vi "2086发送.vi"() -> ()   [LabVIEW 2016, in "数据传输系统-03.lvlib"]
uses:
  <vilib>/Utility/config.llb/Write Key (String).vi
  <vilib>/Utility/config.llb/Read Key (String).vi
  <vilib>/Utility/config.llb/NI_LVConfig.lvlib
panel:
  out "数据发送起始时间":timestamp format="%<%.3X\n%Y/%m/%d>T"
  out "数据拆分":bool
  in  "设备类型":string(combo)="010200"
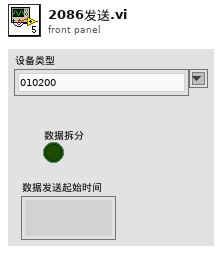
[diagram p1: front panel]
types:
  T1 = cluster{"CODMn":string, "CODCr":string, "DO":string, "铜":string, "PH":string, "氨氮":string, "比电导率":string, "水温":string, "COD":string, "浊度":string, "总氮":string, "总磷":string, "叶绿素a":string, "藻密度":string, "水位":string, "流速":string, "方向":string, "瞬时流量":string, "累积流量":string, "正累积流量":string, "负累积流量":string, "亚硝酸盐":string, "硫化物":string, "ORP":string, "铅":string, "镉":string, "锌":string, "镍":string, "锰":string, "汞":string, "气温":string, "气压":string, "风速":string, "风向":string, "空气温度":string, "相对湿度":string, "分钟雨量":string, "小时雨量":string, "日雨量":string, "累积雨量":string, "盐度":string, "磷酸盐":string, "硝氮":string, "氟化物":string, "挥发酚":string, "氯化物":string, "蓝绿藻":string, "余氯":string, "综合生物毒性":string, "艏向":string, "横摇":string, "纵摇":string, "分层标志":string, "层状态1":string, "层状态2":string, "水平平均流速":string, "流向":string, "北向流速分量":string, "东向流速分量":string, "垂直流速分量":string, "最大波高":string, "最大波周期":string, "1/10波高":string, "1/10波周期":string, "有效波高":string, "有效波周期":string, "平均波高":string, "平均波周期":string, "波向":string, "波个数":string, "水深":string, "X轴流速":string, "Y轴流速":string, "信号强度":string, "电压":string, "悬浮物":string}
  T2 = cluster{"QN":string, "ST":string, "CN":string, "PW":string, "MN":string, "FLAG":string, "PNUM":string, "PNO":string, "CP":string}
  T3 = typedef "LVComboBoxStrsAndValuesArrayTypeDef.ctl" = cluster{"String":string, "Value":string}[]
  T4 = typedef "数据传输系统-03.lvlib/应用环境.ctl" = enum16{"STD", "GB212", "婉仪平台"}
  T5 = cluster{"setini":string, "sysini":string, "hechaini":string, "actualwrite":string, "actualread":string, "datasent":string, "反控命令信息队列":string, "反控与仪器交互":string}
  T6 = cluster{"time1":string, "time2":string, "time3":string, "time4":string, "time5":string, "time6":string, "time7":string, "time8":string, "time9":string, "time10":string, "time11":string, "time12":string, "time13":string, "time14":string, "time15":string, "time16":string, "time17":string, "time18":string, "time19":string, "time20":string, "time21":string, "time22":string, "time23":string, "time24":string, "time25":string, "time26":string, "time27":string, "time28":string, "time29":string, "time30":string, "time31":string, "time32":string, "time33":string, "time34":string, "time35":string, "time36":string, "time37":string, "time38":string, "time39":string, "time40":string, "time41":string, "time42":string, "time43":string, "time44":string, "time45":string, "time46":string, "time47":string, "time48":string, "time49":string, "time50":string, "time51":string, "time52":string, "time53":string, "time54":string, "time55":string, "time56":string, "time57":string, "time58":string, "time59":string, "time60":string, "time61":string, "time62":string, "time63":string, "time64":string, "time65":string, "time66":string, "time67":string, "time68":string, "time69":string, "time70":string, "time71":string, "time72":string, "time73":string, "time74":string, "time75":string, "time76":string}
  T7 = cluster{"水样数据索引[0]":string, "水样数据索引[1]":string, "水样数据索引[2]":string, "水样数据索引[3]":string, "水样数据索引[4]":string, "水样数据索引[5]":string, "水样数据索引[6]":string, "水样数据索引[7]":string, "水样数据索引[8]":string, "水样数据索引[9]":string, "水样数据索引[10]":string, "水样数据索引[11]":string, "水样数据索引[12]":string, "水样数据索引[13]":string, "水样数据索引[14]":string, "水样数据索引[15]":string, "水样数据索引[16]":string, "水样数据索引[17]":string, "水样数据索引[18]":string, "水样数据索引[19]":string, "水样数据索引[20]":string, "水样数据索引[21]":string, "水样数据索引[22]":string, "水样数据索引[23]":string, "水样数据索引[24]":string, "水样数据索引[25]":string, "水样数据索引[26]":string, "水样数据索引[27]":string, "水样数据索引[28]":string, "水样数据索引[29]":string, "水样数据索引[30]":string, "水样数据索引[31]":string, "水样数据索引[32]":string, "水样数据索引[33]":string, "水样数据索引[34]":string, "水样数据索引[35]":string, "水样数据索引[36]":string, "水样数据索引[37]":string, "水样数据索引[38]":string, "水样数据索引[39]":string, "水样数据索引[40]":string, "水样数据索引[41]":string, "水样数据索引[42]":string, "水样数据索引[43]":string, "水样数据索引[44]":string, "水样数据索引[45]":string, "水样数据索引[46]":string, "水样数据索引[47]":string, "水样数据索引[48]":string, "水样数据索引[49]":string, "水样数据索引[50]":string, "水样数据索引[51]":string, "水样数据索引[52]":string, "水样数据索引[53]":string, "水样数据索引[54]":string, "水样数据索引[55]":string, "水样数据索引[56]":string, "水样数据索引[57]":string, "水样数据索引[58]":string, "水样数据索引[59]":string, "水样数据索引[60]":string, "水样数据索引[61]":string, "水样数据索引[62]":string, "水样数据索引[63]":string, "水样数据索引[64]":string, "水样数据索引[65]":string, "水样数据索引[66]":string, "水样数据索引[67]":string, "水样数据索引[68]":string, "水样数据索引[69]":string, "水样数据索引[70]":string, "水样数据索引[71]":string, "水样数据索引[72]":string, "水样数据索引[73]":string, "水样数据索引[74]":string, "水样数据索引[75]":string}
  T8 = typedef "NI_LVConfig.lvlib/Config Data RefNum.ctl" = refnum<k1>
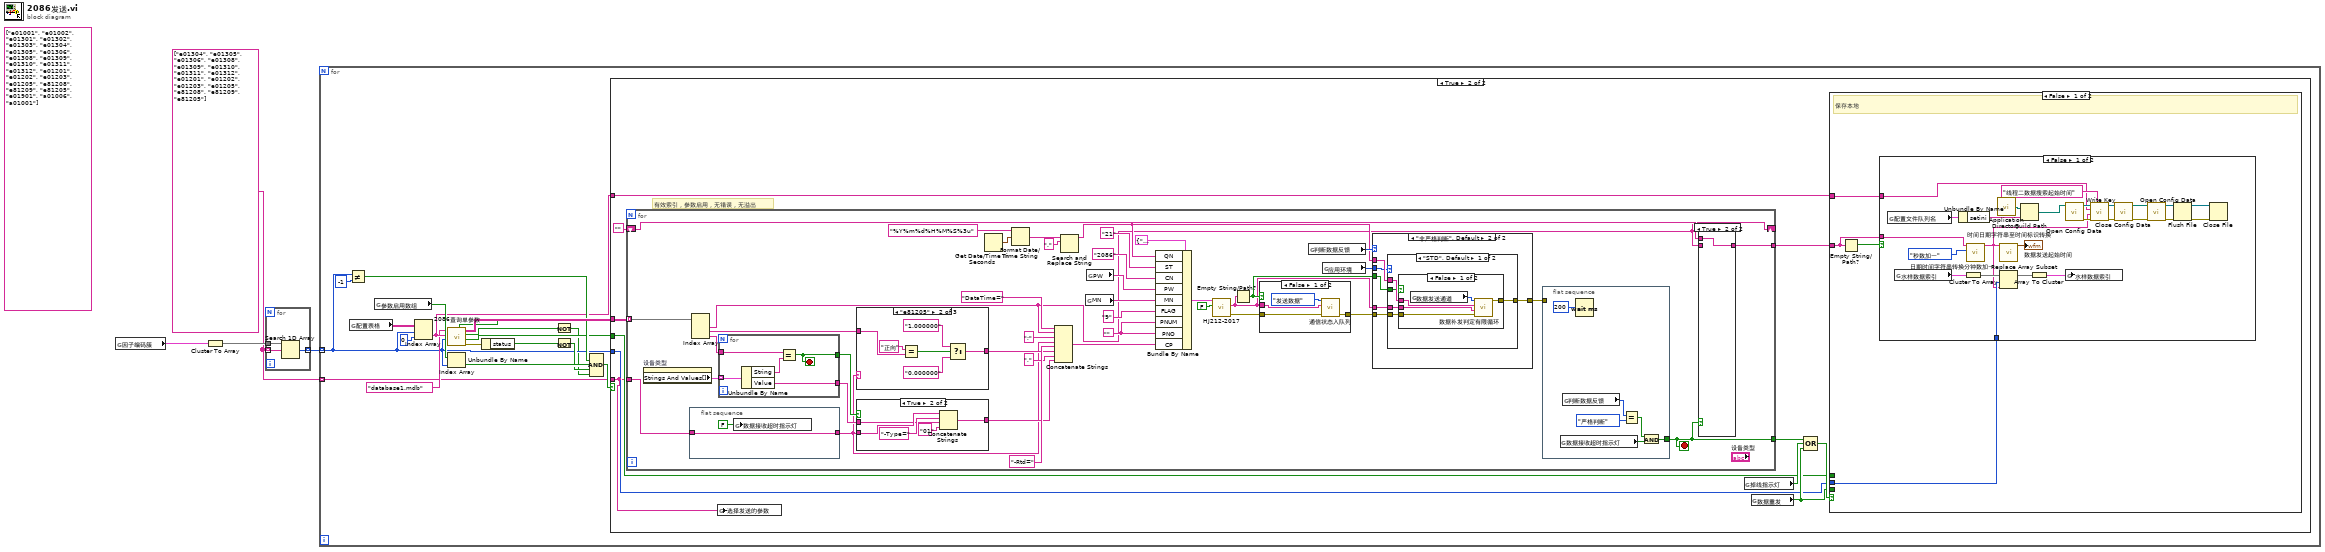
[diagram p0: block diagram]
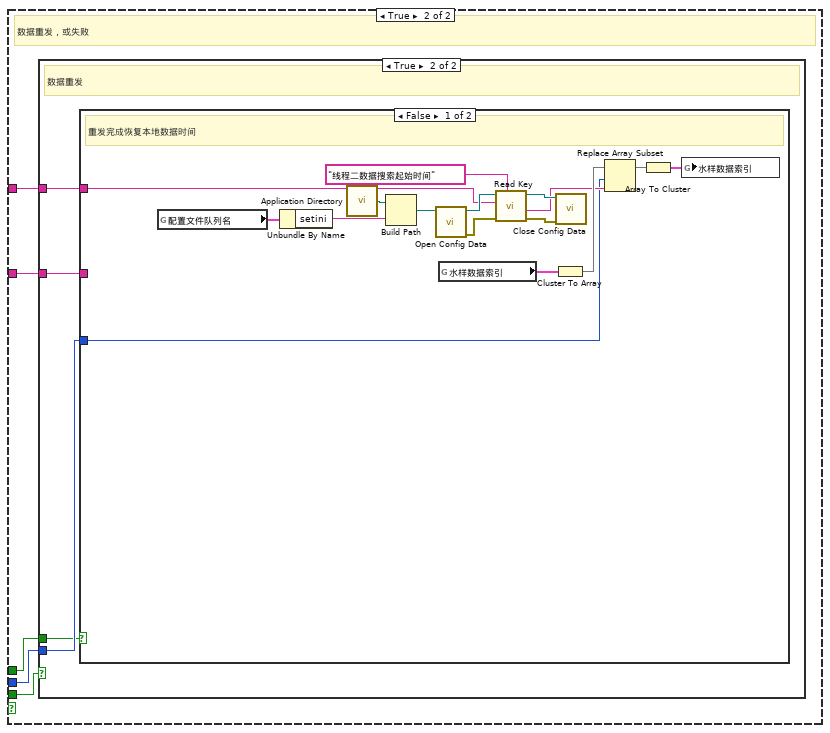
[diagram p4: hidden frame]
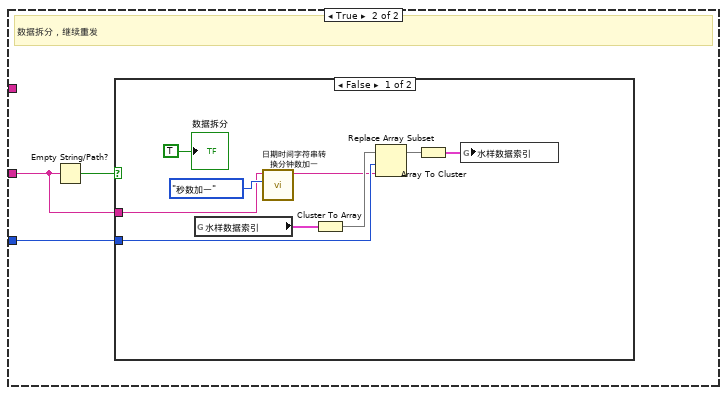
[diagram p6: hidden frame]
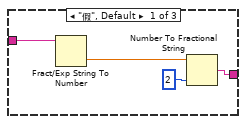
[diagram p9: hidden frame]
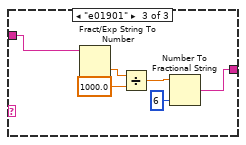
[diagram p10: hidden frame]
diagram:
  (unwired) string[] ["e01001", "e01002", "e01301", "e01302", "e01303", "e01304", "e01305", "e01306", "e01308", "e01309", "e01310", "e01311", "e01312", "e01201", "e01202", "e01203", "e01205", "e81208", "e81209", "e81205", "e01901", "a01006", "a01001"]
  w1 = string[] ["e01304", "e01305", "e01306", "e01308", "e01309", "e01310", "e01311", "e01312", "e01201", "e01202", "e01203", "e01205", "e81208", "e81209", "e81205"]
  n1 = global read "断电保存全局.vi" "因子编码簇"() -> (w4:T1)
  n2 = Cluster To Array(cluster=w4) -> (array=w3:string[])
  n3 = for {
    tunnel: w3 -> [w7]
    tunnel: w1 -> [w6] mode=indexing
    tunnel: [w5] -> w2 mode=indexing
    n4 = Search 1D Array(1D array=w7, element=w6) -> (index of element=w5:i32)  [unwired: 1 in]
  }
  n5 = for {
    tunnel: w2 -> [w11] mode=indexing
    tunnel: w1 -> [w10] mode=indexing
    n6 = Not Equal?(x=w11, y=-1) -> (x != y?=w21:bool)
    n7 = global read "断电保存全局.vi" "配置表格"() -> (w25:string[][])
    n8 = global read "断电保存全局.vi" "参数启用数组"() -> (w22:bool[])
    n9 = Index Array(array=w25, index (row)=w11, index (col)=0 ("y")) -> (element=w19:string)
    n10 = call "2086查询单参数.vi"("索引"=w11, "table"=w19, "database"="database1.mdb") -> ("error out"=w16:errorcluster, "拆分数据"=w17:bool, "database溢出"=w12:bool, "data"=w23:string[][], "有数据"=w8:bool)  [unwired: 4 in]
    n11 = Index Array(array=w22, index=w11) -> (element=w20:bool)
    n12 = Unbundle By Name(w16) -> ("status"=w15:bool)
    n13 = Not(x=w12) -> (.not. x?=w9:bool)
    n14 = Not(x=w15) -> (.not. x?=w14:bool)
    n15 = Compound Arithmetic op=AND ("复合运算")(w8, w21, w20, w14, w9) -> (w13:bool)
    n16 = case shown="True" w13 {
      tunnel: w23 -> [_ w37]
      tunnel: w10 -> [_ w27]
      tunnel: w19 -> [_ w32]
      tunnel: w11 -> [_ w31]
      tunnel: w17 -> [_ w30]
      frame False {
      }
      frame True {
        # "有效索引，参数启用，无错误，无溢出"
        n17 = for {
          tunnel: w37 -> [w104] mode=indexing
          tunnel: w27 -> [w106]
          tunnel: [w110] -> w36
          shift-right: [w105] -> _
          shift-left: "" -> [w109]
          tunnel: [w108] -> w29
          stop <- w110 stop-if-true
          w133 = ""
          n18 = property on="设备类型" class="CmbBox"() -> ("Strings And Values[]"=w126:T3)  [unwired: 2 in, 2 out]
          n19 = flat-sequence {
            tunnel: [w145] -> w107
            tunnel: w106 -> [w145]
            frame #0 {
              n20 = global write "全局 数据发送重叠.vi" "数据接收超时指示灯"(FALSE ("数据接收超时指示灯")) -> ()
            }
          }
          n21 = Index Array(array=w104) -> (element #1=w105:string, element #2=w112:string, element #3=w123:string)  [unwired: 3 in]
          n22 = for {
            tunnel: w126 -> [w200] mode=indexing
            tunnel: w123 -> [w198]
            tunnel: [w197] -> w124
            tunnel: [w196] -> w125
            stop <- w196 stop-if-true
            n23 = Unbundle By Name(w200) -> ("String"=w199:string, "Value"=w197:string)
            n24 = Equal?(x=w198, y=w199) -> (x = y?=w196:bool)
          }
          n25 = case shown="\"e81205\"" w107 {
            tunnel: w112 -> [w149 w157 w159]
            tunnel: [w148 w152 w158] -> w111
            frame "假", Default {
              n26 = Fract/Exp String To Number(string=w149) -> (number=w151:dbl)  [unwired: 3 in, 1 out]
              n27 = Number To Fractional String(number=w151, precision (6)=i16 2 ("精度(6)")) -> (F-format string=w148:string)  [unwired: 2 in]
            }
            frame "e81205" {
              n28 = Equal?(x="正向", y=w157) -> (x = y?=w155:bool)
              n29 = Select(t="1.000000" ("x"), s=w155, f="0.000000" ("x")) -> (s? t:f=w152:string)
            }
            frame "e01901" {
              n30 = Fract/Exp String To Number(string=w159) -> (number=w160:dbl)  [unwired: 3 in, 1 out]
              n31 = Divide(x=w160, y=1000.0) -> (x/y=w162:dbl)
              n32 = Number To Fractional String(number=w162, precision (6)=i16 6 ("精度(6)")) -> (F-format string=w158:string)  [unwired: 2 in]
            }
          }
          n33 = case shown="True" w125 {
            tunnel: w124 -> [_ w193]
            tunnel: w107 -> [_ w195]
            tunnel: [_ w191] -> w121
            frame False {
            }
            frame True {
              n34 = Concatenate Strings(w195, "-Type=" ("格式字符串"), w193, "01" ("字符串")) -> (w191:string)
            }
          }
          n35 = Get Date/Time In Seconds() -> (seconds since 1Jan1904=w141:timestamp)
          n36 = Format Date/Time String(time format string (%c)="%Y%m%d%H%M%S%3u" ("时间格式字符串(%c)"), seconds (now)=w141) -> (date/time string=w140:string)  [unwired: 1 in]
          n37 = Concatenate Strings("DataTime=" ("时间格式字符串(%c)"), w105, ";" ("字符串"), w107, "-Rtd=" ("时间格式字符串(%c)"), w111, "," ("字符串"), w121) -> (w131:string)
          n38 = Search and Replace String(input string=w140, search string="." ("搜索字符串")) -> (result string=w114:string)  [unwired: 6 in, 3 out]
          n39 = global read "断电保存全局.vi" "MN"() -> (w138:string)
          n40 = global read "断电保存全局.vi" "PW"() -> (w137:string)
          n41 = Bundle By Name(cluster=T2 {"QN"="", "ST"="", "CN"="", "PW"="", "MN"="", "FLAG"="", "PNUM"="", "PNO"="", "CP"=""} ("数据块"), "QN"=w114, "ST"="21", "CN"="2086", "PW"=w137, "MN"=w138, "FLAG"="9", "PNUM"=w133, "PNO"=w133, "CP"=w131) -> (w127:T2)
          n42 = call "HJ212-2017.vi"("PWD？"=FALSE, "数据段"=w127) -> ("error out"=w115:errorcluster, "通讯包字符串"=w116:string)  [unwired: 7 in, 1 out]
          n43 = Empty String/Path?(string/path=w116) -> (empty?=w120:bool)
          n44 = case shown="False" w120 {
            tunnel: [w173 w174] -> w118
            tunnel: w115 -> [w172 w174]
            tunnel: w116 -> [w170 _]
            frame False {
              n45 = call "通信状态入队列.vi"("错误输入（无错误）"=w172, "发送报文"=w170, "枚举"=enum16{"打开连接", "发送数据", "读取数据", "数据处理", "关闭连接"}."发送数据") -> ("错误输出"=w173:errorcluster)  [unwired: 8 in]
            }
            frame True {
            }
          }
          n46 = global read "断电保存全局.vi" "判断数据反馈"() -> (w117:enum16{"非严格判断", "严格判断", "不判断"})
          n47 = global read "断电保存全局.vi" "应用环境"() -> (w119:T4)
          n48 = case shown="\"非严格判断\", Default" w117 {
            tunnel: w116 -> [_ w180]
            tunnel: w118 -> [_ w179]
            tunnel: w114 -> [_ w178]
            tunnel: w119 -> [_ w177]
            tunnel: w120 -> [_ w176]
            tunnel: [_ w175] -> w113
            frame "不判断" {
            }
            frame "非严格判断", Default {
              n49 = case shown="\"STD\", Default" w177 {
                tunnel: w180 -> [w183 _]
                tunnel: w179 -> [w185 _]
                tunnel: w178 -> [w184 _]
                tunnel: w176 -> [w182 _]
                tunnel: [w181 _] -> w175
                frame "STD", Default {
                  n50 = case shown="False" w182 {
                    tunnel: w185 -> [w190 _]
                    tunnel: w184 -> [w188 _]
                    tunnel: w183 -> [w187 _]
                    tunnel: [w186 _] -> w181
                    frame False {
                      n51 = global read "断电保存全局.vi" "数据发送通道"() -> (w189:enum16{"TCP", "VISA"})
                      n52 = call "数据补发判定有限循环.vi"("错误输入（无错误）"=w190, "数据输入"=w187, "QN"=w188, "数据发送通道"=w189) -> ("error out"=w186:errorcluster)  [unwired: 7 in]
                    }
                    frame True {
                    }
                  }
                }
                frame "GB212" {
                }
              }
            }
          }
          n53 = flat-sequence {
            tunnel: w113 -> [_]
            tunnel: [w166] -> w110
            frame #0 {
              n54 = global read "全局 数据发送重叠.vi" "数据接收超时指示灯"() -> (w169:bool)
              n55 = global read "断电保存全局.vi" "判断数据反馈"() -> (w167:enum16{"非严格判断", "严格判断", "不判断"})
              n56 = Wait (ms)(milliseconds to wait=u32 200 ("等待时间（毫秒）")) -> ()  [unwired: 1 out]
              n57 = Equal?(x=w167, y=enum16{"非严格判断", "严格判断", "不判断"}."严格判断") -> (x = y?=w164:bool)
              n58 = And(x=w164, y=w169) -> (x .and. y?=w166:bool)
            }
          }
          n59 = case shown="True" w110 {
            tunnel: w109 -> [_ w147]
            tunnel: [w146 w147] -> w108
            tunnel: w105 -> [w146 _]
            frame False {
            }
            frame True {
            }
          }
        }
        n60 = global write "全局 水样时间.vi" "选择发送的参数"(w27) -> ()
        n61 = global read "全局 数据发送重叠.vi" "掉线指示灯"() -> (w35:bool)
        n62 = global read "断电保存全局.vi" "数据重发"() -> (w33:bool)
        n63 = Compound Arithmetic op=OR ("复合运算")(w36, w35, w33) -> (w34:bool)
        n64 = case shown="False" w34 {
          tunnel: w29 -> [w38 w67]
          tunnel: w31 -> [w40 w69]
          tunnel: w32 -> [w41 w71]
          tunnel: w33 -> [_ w70]
          tunnel: w30 -> [_ w68]
          frame False {
            # "保存本地"
            n65 = Empty String/Path?(string/path=w38) -> (empty?=w39:bool)
            n66 = case shown="False" w39 {
              tunnel: w41 -> [w59 _]
              tunnel: w40 -> [w53 _]
              tunnel: w38 -> [w48 _]
              frame False {
                n67 = global read "全局1.vi" "配置文件队列名"() -> (w49:T5)
                n68 = global read "全局 水样时间.vi" "水样数据索引"() -> (w54:T6)
                n69 = Unbundle By Name(w49) -> ("setini"=w50:string)
                n70 = Cluster To Array(cluster=w54) -> (array=w55:string[])
                n71 = call "日期时间字符串转换分钟数加一.vi"("枚举"=enum16{"分钟数加一", "秒数加一", "小时数加一"}."秒数加一", "data[0]"=w48) -> ("日期/时间字符串"=w52:string)  [unwired: 9 in]
                n72 = call <vilib>:"Application Directory.vi"() -> ("Application Directory"=w60:path)
                n73 = call "时间日期字符串至时间标识转换.vi"("时间日期字符串"=w52) -> ("时间标识"=→"数据发送起始时间":timestamp)  [unwired: 10 in]
                n74 = Replace Array Subset(array=w55, new element=w52, index=w53) -> (w56:string[])
                n75 = Build Path(base path=w60, name or relative path=w50) -> (appended path=w61:path)
                n76 = Array To Cluster(array=w56) -> (cluster=w57:T7)
                n77 = call <vilib>:"Open Config Data.vi"("configuration file path"=w61) -> ("error out"=w63:errorcluster, "refnum"=w62:T8)  [unwired: 8 in, 1 out]
                n78 = global write "全局 水样时间.vi" "水样数据索引"(w57) -> ()
                n79 = call-poly <vilib>:"Write Key.vi"("section"="线程二数据搜索起始时间", "error in (no error)"=w63, "value"=w52, "key"=w59, "refnum"=w62) -> ("error out"=w65:errorcluster, "refnum out"=w64:T8)  [unwired: 4 in, 1 out]
                n80 = call <vilib>:"Close Config Data.vi"("error in (no error)"=w65, "refnum"=w64) -> ("error out"=w47:errorcluster, "file path"=w46:path)  [unwired: 8 in]
                n81 = call <vilib>:"Open Config Data.vi"("error in (no error)"=w47, "configuration file path"=w46) -> ("error out"=w45:errorcluster, "refnum"=w44:T8)  [unwired: 7 in, 1 out]
                n82 = Flush File(refnum=w44, error in=w45) -> (refnum out=w43:T8, error out=w42:errorcluster)
                n83 = Close File(refnum=w43, error in=w42) -> ()  [unwired: 2 out]
              }
              frame True {
              }
            }
          }
          frame True {
            # "数据重发，或失败"
            n84 = case shown="True" w70 {
              tunnel: w71 -> [_ w75]
              tunnel: w69 -> [_ w74]
              tunnel: w68 -> [_ w73]
              tunnel: w67 -> [_ w72]
              frame False {
                # "数据发送失败"
              }
              frame True {
                # "数据重发"
                n85 = case shown="False" w73 {
                  tunnel: w75 -> [w79 _]
                  tunnel: w74 -> [w77 w94]
                  tunnel: w72 -> [_ w92]
                  frame False {
                    # "重发完成恢复本地数据时间"
                    n86 = global read "全局1.vi" "配置文件队列名"() -> (w76:T5)
                    n87 = Unbundle By Name(w76) -> ("setini"=w86:string)
                    n88 = call <vilib>:"Application Directory.vi"() -> ("Application Directory"=w80:path)
                    n89 = Build Path(base path=w80, name or relative path=w86) -> (appended path=w81:path)
                    n90 = call <vilib>:"Open Config Data.vi"("configuration file path"=w81) -> ("error out"=w87:errorcluster, "refnum"=w82:T8)  [unwired: 8 in, 1 out]
                    n91 = global read "全局 水样时间.vi" "水样数据索引"() -> (w88:T6)
                    n92 = call-poly <vilib>:"Read Key.vi"("section"="线程二数据搜索起始时间", "error in (no error)"=w87, "key"=w79, "refnum"=w82) -> ("error out"=w85:errorcluster, "value"=w78:string, "refnum out"=w84:T8)  [unwired: 4 in, 1 out]
                    n93 = Cluster To Array(cluster=w88) -> (array=w89:string[])
                    n94 = call <vilib>:"Close Config Data.vi"("error in (no error)"=w85, "refnum"=w84) -> ()  [unwired: 8 in, 2 out]
                    n95 = Replace Array Subset(array=w89, new element=w78, index=w77) -> (w90:string[])
                    n96 = Array To Cluster(array=w90) -> (cluster=w91:T7)
                    n97 = global write "全局 水样时间.vi" "水样数据索引"(w91) -> ()
                  }
                  frame True {
                    # "数据拆分，继续重发"
                    n98 = Empty String/Path?(string/path=w92) -> (empty?=w93:bool)
                    n99 = case shown="False" w93 {
                      tunnel: w94 -> [w98 _]
                      tunnel: w92 -> [w95 _]
                      frame False {
                        n100 = global read "全局 水样时间.vi" "水样数据索引"() -> (w99:T6)
                        n101 = call "日期时间字符串转换分钟数加一.vi"("枚举"=enum16{"分钟数加一", "秒数加一", "小时数加一"}."秒数加一", "data[0]"=w95) -> ("日期/时间字符串"=w97:string)  [unwired: 9 in]
                        n102 = Cluster To Array(cluster=w99) -> (array=w100:string[])
                        n103 = Replace Array Subset(array=w100, new element=w97, index=w98) -> (w101:string[])
                        n104 = Array To Cluster(array=w101) -> (cluster=w102:T7)
                        n105 = global write "全局 水样时间.vi" "水样数据索引"(w102) -> ()
                        "数据拆分" <- TRUE
                      }
                      frame True {
                      }
                    }
                  }
                }
              }
            }
          }
        }
      }
    }
  }
